vi "FMI_CH2.vi"(2 "Accel":i32=1000, 3 "Direction":enum16{"Forward", "Reverse"}(ring), 4 "RPM":i32=375, 6 "Strokes":i32=3, 7 "Home Pump":bool) -> (0 "FMI_Disconnect":bool=TRUE)   [LabVIEW 2019]
uses:
  C:/Users/MUSE_V2/Desktop/CLIO/ConfigFiles/FMI_labview/FMI_LIB.dll
  ConfigFiles/FMI_labview/FMI_LIB.dll
panel:
  out "seconds before timer start":dbl
  out "Pumping Progress":dbl(slide)=1.0091556705865854 scale=0.0..1.0
  out "Step Completion (%)":dbl=100.91556705865854
  out "Stroke#":dbl format="%#_4g"
  in  "ProgressBar?":bool
  out "Pump Start":bool=TRUE
  out "Pump Runtime (s)":dbl=2.0094395102393197
  out "FMI_Connect":bool
  in  "VISA resource name":refnum<visa-resource-name>="COM5"
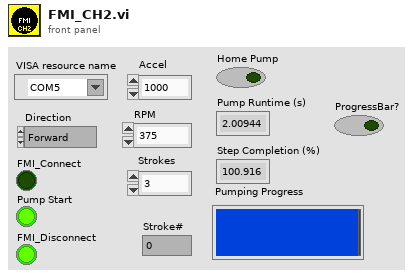
[diagram p1: front panel]
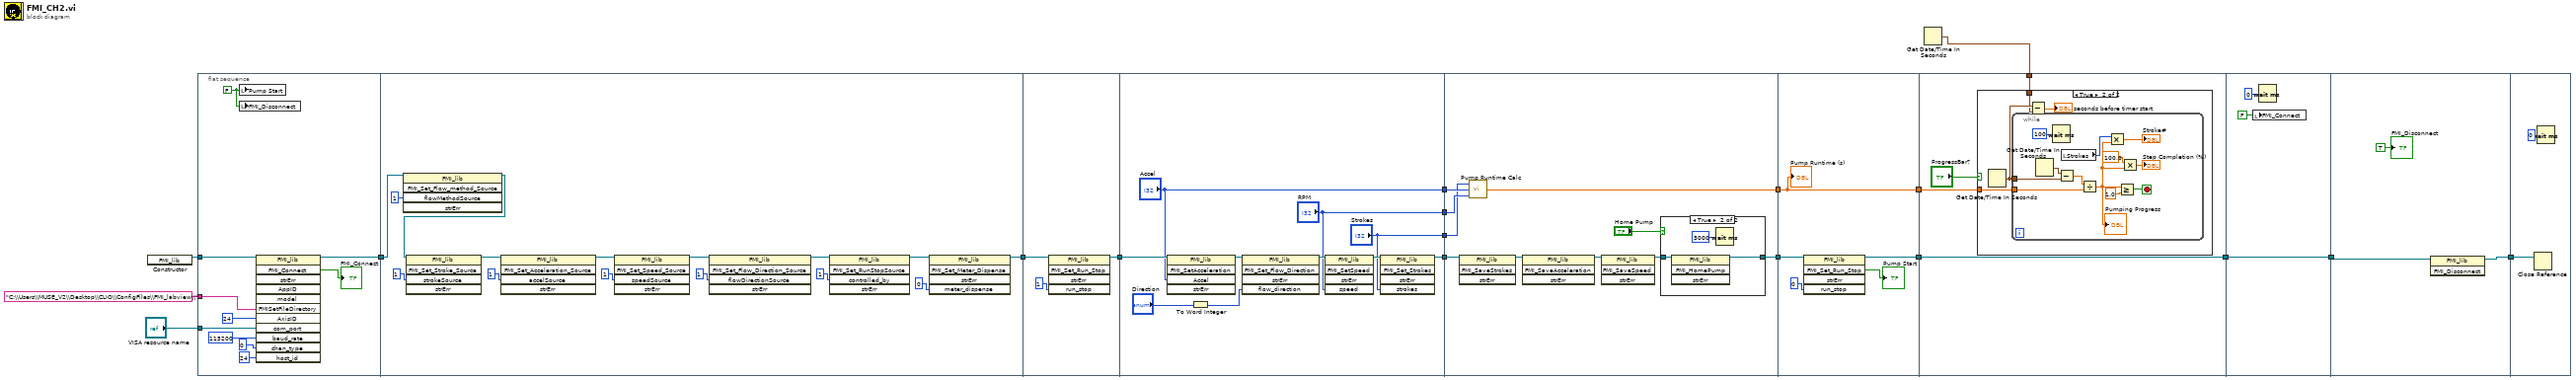
[diagram p0: block diagram]
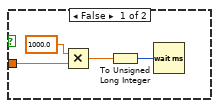
[diagram p3: hidden frame]
diagram:
  n1 = constructor class="FMI_lib"() -> (reference out=w6:refnum<k24>)  [unwired: 3 in, 2 out]
  n2 = flat-sequence {
    tunnel: [w25] -> w18
    tunnel: w6 -> [w28]
    tunnel: "C:\\Users\\MUSE_V2\\Desktop\\CLIO\\ConfigFiles\\FMI_labview\\" ("Path to setup files") -> [w26]
    tunnel: "VISA resource name" -> [w22]
    tunnel: w18 -> [w31]
    tunnel: [w32] -> w17
    tunnel: w17 -> [w45]
    tunnel: [w44] -> w16
    tunnel: w16 -> [w56]
    tunnel: [w52] -> w15
    tunnel: ["Accel"] -> w14
    tunnel: ["RPM"] -> w13
    tunnel: ["Strokes"] -> w12
    tunnel: w15 -> [w66]
    tunnel: [w58] -> w11
    tunnel: w14 -> [w63]
    tunnel: w13 -> [w62]
    tunnel: w12 -> [w61]
    tunnel: [w60] -> w10
    tunnel: w11 -> [w74]
    tunnel: [w73] -> w9
    tunnel: [w71] -> w8
    tunnel: w10 -> [w71]
    tunnel: [w79] -> w7
    tunnel: w9 -> [w79]
    tunnel: w8 -> [w78]
    tunnel: w2 -> [w76]
    tunnel: w7 -> [w100]
    tunnel: [w100] -> w1
    tunnel: [w105] -> w3
    tunnel: w1 -> [w103]
    tunnel: w3 -> [w107]
    frame #0 {
      w23 = FALSE
      n3 = local write "Pump Start"(w23) -> ()
      n4 = local write "FMI_Disconnect"(w23) -> ()
      n5 = invoke class="FMI_lib" method="FMI_Connect"(reference=w28, "FMISetFileDirectory"=w26, "AxisID"=u8 24, "com_port"=w22, "baud_rate"=u32 115200, "chan_type"=u8 0, "host_id"=u8 24) -> (reference out=w25:refnum<k24>, "FMI_Connect"=→"FMI_Connect":bool)  [unwired: 5 in, 10 out]
    }
    frame #1 {
      n6 = invoke class="FMI_lib" method="FMI_Set_Flow_method_Source"(reference=w31, "flowMethodSource"=i16 1) -> (reference out=w30:refnum<k24>)  [unwired: 3 in, 4 out]
      n7 = invoke class="FMI_lib" method="FMI_Set_Stroke_Source"(reference=w30, "strokeSource"=i16 1) -> (reference out=w39:refnum<k24>)  [unwired: 3 in, 4 out]
      n8 = invoke class="FMI_lib" method="FMI_Set_Acceleration_Source"(reference=w39, "accelSource"=i16 1) -> (reference out=w38:refnum<k24>)  [unwired: 3 in, 4 out]
      n9 = invoke class="FMI_lib" method="FMI_Set_Speed_Source"(reference=w38, "speedSource"=i16 1 ("strokeSource")) -> (reference out=w37:refnum<k24>)  [unwired: 3 in, 4 out]
      n10 = invoke class="FMI_lib" method="FMI_Set_Flow_Direction_Source"(reference=w37, "flowDirectionSource"=i16 1) -> (reference out=w36:refnum<k24>)  [unwired: 3 in, 4 out]
      n11 = invoke class="FMI_lib" method="FMI_Set_RunStopSource"(reference=w36, "controlled_by"=i16 1) -> (reference out=w33:refnum<k24>)  [unwired: 3 in, 4 out]
      n12 = invoke class="FMI_lib" method="FMI_Set_Meter_Dispense"(reference=w33, "meter_dispense"=i16 0) -> (reference out=w32:refnum<k24>)  [unwired: 3 in, 4 out]
    }
    frame #2 {
      n13 = invoke class="FMI_lib" method="FMI_Set_Run_Stop"(reference=w45, "run_stop"=i16 1) -> (reference out=w44:refnum<k24>)  [unwired: 3 in, 4 out]
    }
    frame #3 {
      n14 = invoke class="FMI_lib" method="FMI_SetAcceleration"(reference=w56, "Accel"="Accel") -> (reference out=w55:refnum<k24>)  [unwired: 3 in, 4 out]
      n15 = To Word Integer(number="Direction") -> (16bit integer=w47:i16)
      n16 = invoke class="FMI_lib" method="FMI_Set_Flow_Direction"(reference=w55, "flow_direction"=w47) -> (reference out=w54:refnum<k24>)  [unwired: 3 in, 4 out]
      n17 = invoke class="FMI_lib" method="FMI_SetSpeed"(reference=w54, "speed"="RPM") -> (reference out=w53:refnum<k24>)  [unwired: 3 in, 4 out]
      n18 = invoke class="FMI_lib" method="FMI_Set_Strokes"(reference=w53, "strokes"="Strokes") -> (reference out=w52:refnum<k24>)  [unwired: 3 in, 4 out]
    }
    frame #4 {
      n19 = invoke class="FMI_lib" method="FMI_SaveStrokes"(reference=w66) -> (reference out=w65:refnum<k24>)  [unwired: 3 in, 3 out]
      n20 = call "Pump Runtime Calc.vi"("RPM"=w62, "Accel"=w63, "Strokes"=w61) -> ("Pump Runtime (s)"=w60:dbl)
      n21 = invoke class="FMI_lib" method="FMI_SaveAcceleration"(reference=w65) -> (reference out=w64:refnum<k24>)  [unwired: 3 in, 3 out]
      n22 = invoke class="FMI_lib" method="FMI_SaveSpeed"(reference=w64) -> (reference out=w59:refnum<k24>)  [unwired: 3 in, 3 out]
      n23 = case shown="True" "Home Pump" {
        tunnel: w59 -> [w67 w70]
        tunnel: [w67 w69] -> w58
        frame False {
        }
        frame True {
          n24 = invoke class="FMI_lib" method="FMI_HomePump"(reference=w70) -> (reference out=w69:refnum<k24>)  [unwired: 3 in, 3 out]
          n25 = Wait (ms)(milliseconds to wait=u32 3000) -> ()  [unwired: 1 out]
        }
      }
    }
    frame #5 {
      n26 = invoke class="FMI_lib" method="FMI_Set_Run_Stop"(reference=w74, "run_stop"=i16 0) -> (reference out=w73:refnum<k24>, "FMI_Set_Run_Stop"=→"Pump Start":bool)  [unwired: 3 in, 3 out]
      "Pump Runtime (s)" <- w71
    }
    frame #6 {
      n27 = case shown="True" "ProgressBar?" {
        tunnel: w78 -> [w83 w87]
        tunnel: w76 -> [_ w85]
        frame False {
          n28 = Multiply(x=1000.0, y=w83) -> (x*y=w81:dbl)
          n29 = To Unsigned Long Integer(number=w81) -> (unsigned 32bit integer=w80:u32)
          n30 = Wait (ms)(milliseconds to wait=w80) -> ()  [unwired: 1 out]
        }
        frame True {
          n31 = Get Date/Time In Seconds() -> (seconds since 1Jan1904=w86:timestamp)
          n32 = while {
            tunnel: w86 -> [w97]
            tunnel: w87 -> [w94]
            stop <- w98 stop-if-true
            n33 = Get Date/Time In Seconds() -> (seconds since 1Jan1904=w95:timestamp)
            n34 = Wait (ms)(milliseconds to wait=u32 100) -> ()  [unwired: 1 out]
            n35 = Subtract(x=w95, y=w97) -> (x-y=w96:dbl)
            n36 = local read "Strokes"() -> (w89:i32)
            n37 = Divide(x=w96, y=w94) -> (x/y=w90:dbl)
            "Pumping Progress" <- w90
            n38 = Multiply(x=w89, y=w90) -> (x*y=→"Stroke#":dbl)
            n39 = Greater Or Equal?(x=w90, y=1.0) -> (x >= y?=w98:bool)
            n40 = Multiply(x=100.0, y=w90) -> (x*y=→"Step Completion (%)":dbl)
          }
          n41 = Subtract(x=w86, y=w85) -> (x-y=→"seconds before timer start":dbl)
        }
      }
    }
    frame #7 {
      n42 = local write "FMI_Connect"(FALSE) -> ()
      n43 = Wait (ms)(milliseconds to wait=u32 0) -> ()  [unwired: 1 out]
    }
    frame #8 {
      n44 = invoke class="FMI_lib" method="FMI_Disconnect"(reference=w103) -> (reference out=w105:refnum<k24>)  [unwired: 2 in, 2 out]
      "FMI_Disconnect" <- TRUE
    }
    frame #9 {
      n45 = Close Reference(reference=w107) -> ()  [unwired: 1 in, 1 out]
      n46 = Wait (ms)(milliseconds to wait=u32 0) -> ()  [unwired: 1 out]
    }
  }
  n47 = Get Date/Time In Seconds() -> (seconds since 1Jan1904=w2:timestamp)
